vi "Get Ending.vi"(8 "error in (no error)":errorcluster, 11 "Range in":refnum<class "Range.lvclass">) -> (0 "error out":errorcluster, 2 "Ending out":refnum<class "Data.lvclass">, 3 "Range out":refnum<class "Range.lvclass">)   [LabVIEW 2012, in "MDSplus.lvlib" / "Range.lvclass"]
uses:
  <vilib>/MDSplus/Classes/Data_Class/Compound_Class/Range_Class/Range.lvclass
  <vilib>/MDSplus/Classes/Data_Class/Data.lvclass
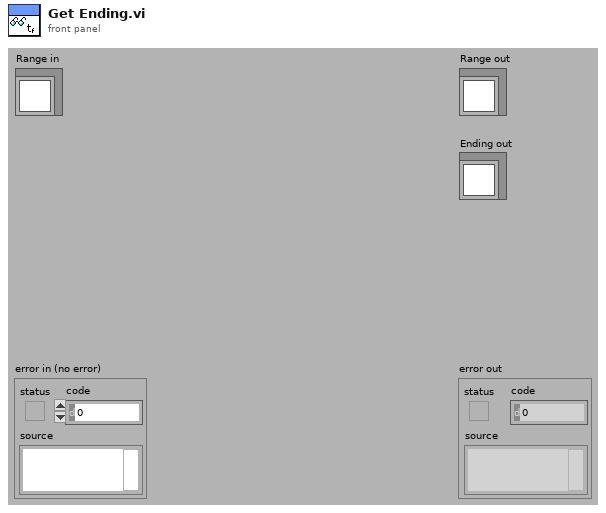
[diagram p1: front panel]
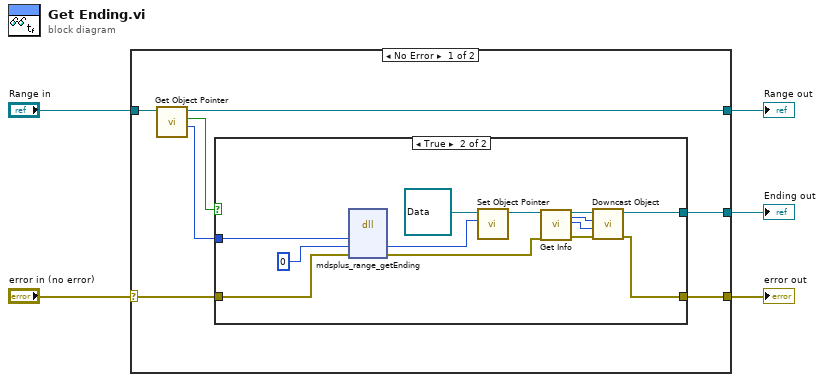
[diagram p0: block diagram]
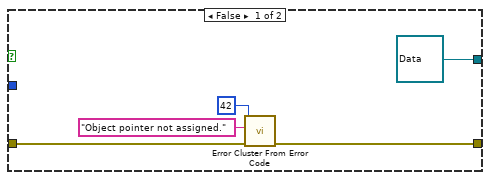
[diagram p2: hidden frame]
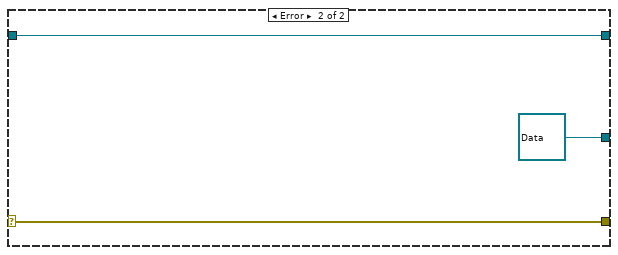
[diagram p3: hidden frame]
diagram:
  n1 = case shown="No Error" "error in (no error)" {
    selector: "error in (no error)" -> [w8 w33]
    tunnel: [w7 w33] -> w4
    tunnel: [w6 w32] -> w2
    tunnel: "Range in" -> [w11 w32]
    tunnel: [w12 refnum<class "Data.lvclass"> refnum ("Data out")] -> w1
    frame No Error {
      n2 = call-dynamic "Get Object Pointer.vi"("Data in"=w11) -> ("Object Pointer"=w9:i64, "Assigned object pointer?"=w10:bool, "Data out"=w6:refnum<class "Range.lvclass">)  [unwired: 8 in]
      n3 = case shown="True" w10 {
        tunnel: [refnum<class "Data.lvclass"> refnum ("Data out") w22] -> w12
        tunnel: w9 -> [_ w21]
        tunnel: w8 -> [w14 w19]
        tunnel: [w13 w18] -> w7
        frame False {
          n4 = call <vilib>:"Error Cluster From Error Code.vi"("error in (no error)"=w14, "error message (\"\")"="Object pointer not assigned." ("error message (\"\")"), "error code (0)"=42) -> ("error out"=w13:errorcluster)  [unwired: 6 in]
        }
        frame True {
          n5 = dll-call lib="MDSobjectsLVShr" fn="mdsplus_range_getEnding"("lvRangePtr"=w21, "lvDataPtrOut"=i64 0, "error"=w19) -> ("lvDataPtrOut"=w28:i64, "error"=w20:errorcluster)  [unwired: 5 in, 2 out]
          n6 = call-dynamic "Set Object Pointer.vi"("Object Pointer"=w28, "Data in"=refnum<class "Data.lvclass"> refnum ("Data.lvclass")) -> ("Data out"=w27:refnum<class "Data.lvclass">)  [unwired: 9 in]
          n7 = call-dynamic "Get Info.vi"("Data in"=w27, "error in (no error)"=w20) -> ("Data out"=w26:refnum<class "Data.lvclass">, "Class type out"=w25:u8, "Data type out"=w24:u8, "error out"=w23:errorcluster)  [unwired: 12 in, 2 out]
          n8 = call <vilib>:"Downcast Object.vi"("error in (no error)"=w23, "Data Type"=w24, "Class Type"=w25, "Data in"=w26) -> ("error out"=w18:errorcluster, "Data out"=w22:refnum<class "Data.lvclass">)  [unwired: 6 in]
        }
      }
    }
    frame Error {
    }
  }
  "error out" <- w4
  "Range out" <- w2
  "Ending out" <- w1
